vi "seriesInfo.get.vi"(11 "ComicVine_class in":refnum<class "series_class.lvclass">) -> (2 "seriesInfo":T1, 3 "ComicVine_class out":refnum<class "series_class.lvclass">)   [LabVIEW 2024, in "series_class.lvclass"]
uses:
  series_class.lvclass
  definitions/seriesInfo.ctl
  series_class.lvclass/series_class.ctl
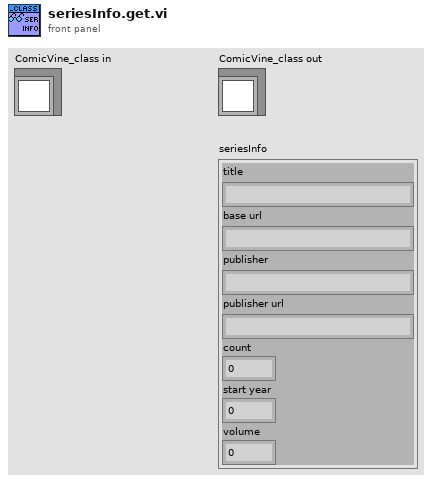
[diagram p1: front panel]
types:
  T1 = typedef "seriesInfo.ctl" = cluster{"title":string, "base url":string, "publisher":string, "publisher url":string, "count":i32, "start year":i32, "volume":i32}
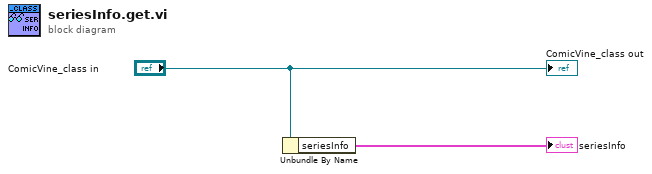
[diagram p0: block diagram]
diagram:
  n1 = Unbundle By Name("ComicVine_class in") -> ("seriesInfo"=→"seriesInfo":T1)
  "ComicVine_class out" <- "ComicVine_class in"
